vi "libssh2_hostkey_hash.vi"(8 "error in (no error)":errorcluster, 10 "hash type":T1=enum."SHA1", 11 "session":T2) -> (0 "error out":errorcluster, 2 "hash":u8[](array[numeric]))   [LabVIEW 2013, in "libssh2.lvlib"]
doc: "Get the hash of the remote host's public key."
uses:
  libssh2.lvlib
  Session Refnum.ctl
  Host Key Hash Type.ctl
  Not A Session.vi
  <vilib>/Utility/error.llb/Error Cluster From Error Code.vi
  Global Settings.vi
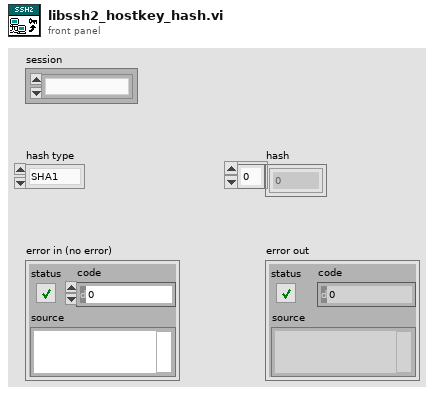
[diagram p1: front panel]
types:
  T1 = typedef "libssh2.lvlib/Host Key Hash Type.ctl" = enum16{"MD5", "SHA1", "SHA256"}
  T2 = typedef "libssh2.lvlib/Session Refnum.ctl" = refnum<k1>
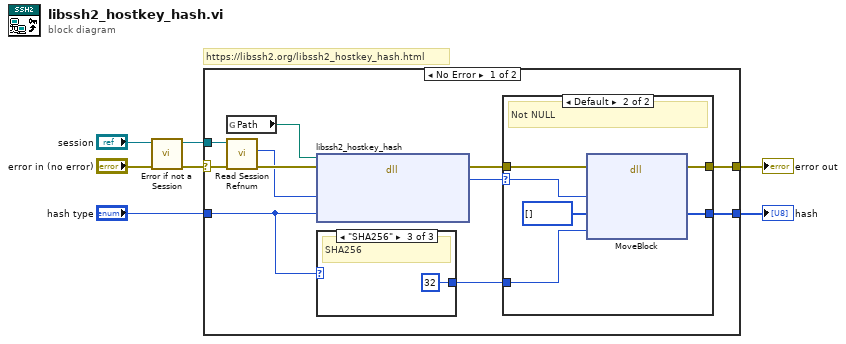
[diagram p0: block diagram]
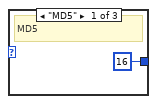
[diagram p3: hidden frame]
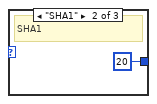
[diagram p4: hidden frame]
diagram:
  # "https://libssh2.org/libssh2_hostkey_hash.html"
  n1 = call "Error if not a Session.vi"("error in (no error)"="error in (no error)", "session"="session") -> ("error out"=w3:errorcluster, "session out"=w1:T2)  [unwired: 8 in]
  n2 = case shown="No Error" w3 {
    selector: w3 -> [w18 w29]
    tunnel: "hash type" -> [w16 _]
    tunnel: [w17 w29] -> w6
    tunnel: w1 -> [w14 _]
    tunnel: [w15 _] -> w4
    frame No Error {
      n3 = global read "Global Settings.vi" "Path"() -> (w9:path)
      n4 = call "Read Session Refnum.vi"("error in (no error)"=w18, "session"=w14) -> ("error out"=w13:errorcluster, "LIBSSH2_SESSION*"=w12:u64)  [unwired: 5 in, 3 out]
      n5 = dll-call lib="?" fn="libssh2_hostkey_hash"(path in=w9, error in=w13, "session"=w12, "hash_type"=w16) -> (error out=w11:errorcluster, "return value"=w8:u64)  [unwired: 3 in, 1 out]
      n6 = case shown="\"SHA256\"" w16 {
        tunnel: [i64 16 ("dimension size") i64 20 ("dimension size") i64 32 ("dimension size")] -> w10
        frame "MD5" {
          # "MD5"
        }
        frame "SHA1" {
          # "SHA1"
        }
        frame "SHA256" {
          # "SHA256"
        }
      }
      n7 = case shown="Default" w8 {
        selector: w8 -> [_ w20]
        tunnel: w11 -> [w19 w25]
        tunnel: [w19 w24] -> w17
        tunnel: w10 -> [_ w22]
        tunnel: [_ w21] -> w15
        frame 0 {
          # "NULL"
        }
        frame Default {
          # "Not NULL"
          n8 = dll-call lib="LabVIEW" fn="MoveBlock"(error in=w25, "ps"=w20, "pd"=u8[] [], "size"=w22) -> (error out=w24:errorcluster, "pd"=w21:u8[])  [unwired: 5 in, 1 out]
        }
      }
    }
    frame Error {
    }
  }
  "error out" <- w6
  "hash" <- w4
